vi "Kinect Analyze Particle.vi"(0 "Particle Mask In":T2, 5 "Extracted Mouse Image":T2, 7 "Height Threshold":dbl=100.0 format="%0.2f", 9 "Mouse Orientation":i32, 11 "error in":errorcluster) -> (4 "Mouse Data":T1, 15 "error out":errorcluster)   [LabVIEW 2011]
uses:
  <vilib>/vision/Image Controls.llb/IMAQ Image.ctl
  Mouse Data Cluster.ctl
  <vilib>/vision/NI_Vision_Development_Module.lvlib
panel:
  in  "Width of Band to \nCalculate Average Contour":i32=10
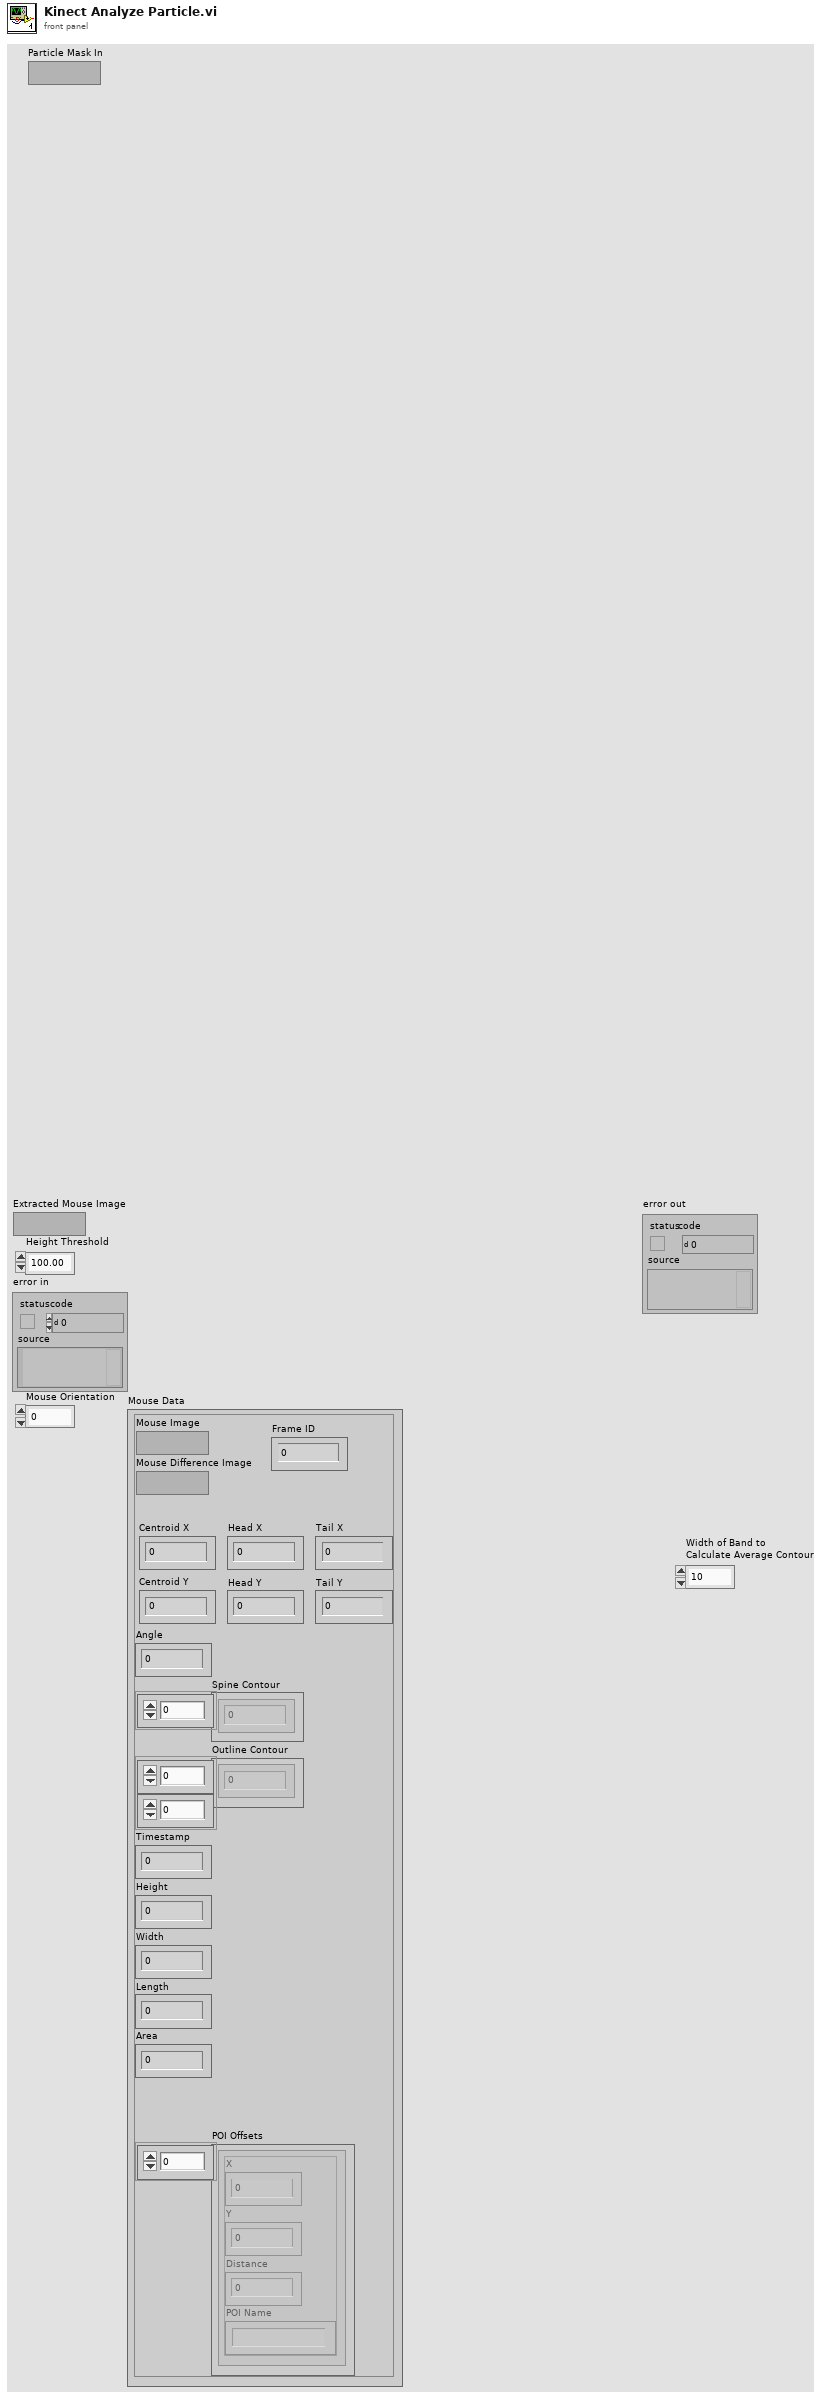
[diagram p1: front panel]
types:
  T1 = typedef "Mouse Data Cluster.ctl" = cluster{"Mouse Image":T2, "Mouse Difference Image":T2, "Angle":i32, "Spine Contour":i32[], "Outline Contour":i32[][], "Timestamp":dbl, "Height":i32, "Width":i32, "Length":i32, "Area":sgl, "POI Offsets":cluster{"X":i32, "Y":i32, "Distance":i32, "POI Name":string}[], "Frame ID":i16, "Centroid X":i32, "Centroid Y":i32, "Head X":i32, "Head Y":i32, "Tail X":i32, "Tail Y":i32}
  T2 = typedef "IMAQ Image.ctl" = refnum<image>
  T3 = typedef "Particle Parameters" = i32
  T4 = typedef "ROI Descriptor" = cluster{"Global Rectangle":i32[], "Contours":cluster{"ID":enum32{"External", "Internal"}, "Type":u32, "Coordinates":i32[]}[]}
  T5 = cluster{"ID":enum32{"External", "Internal"}, "Type":u32, "Coordinates":i32[]}[]
  T6 = cluster{"ID":enum32{"External", "Internal"}, "Type":u32, "Coordinates":i32[]}
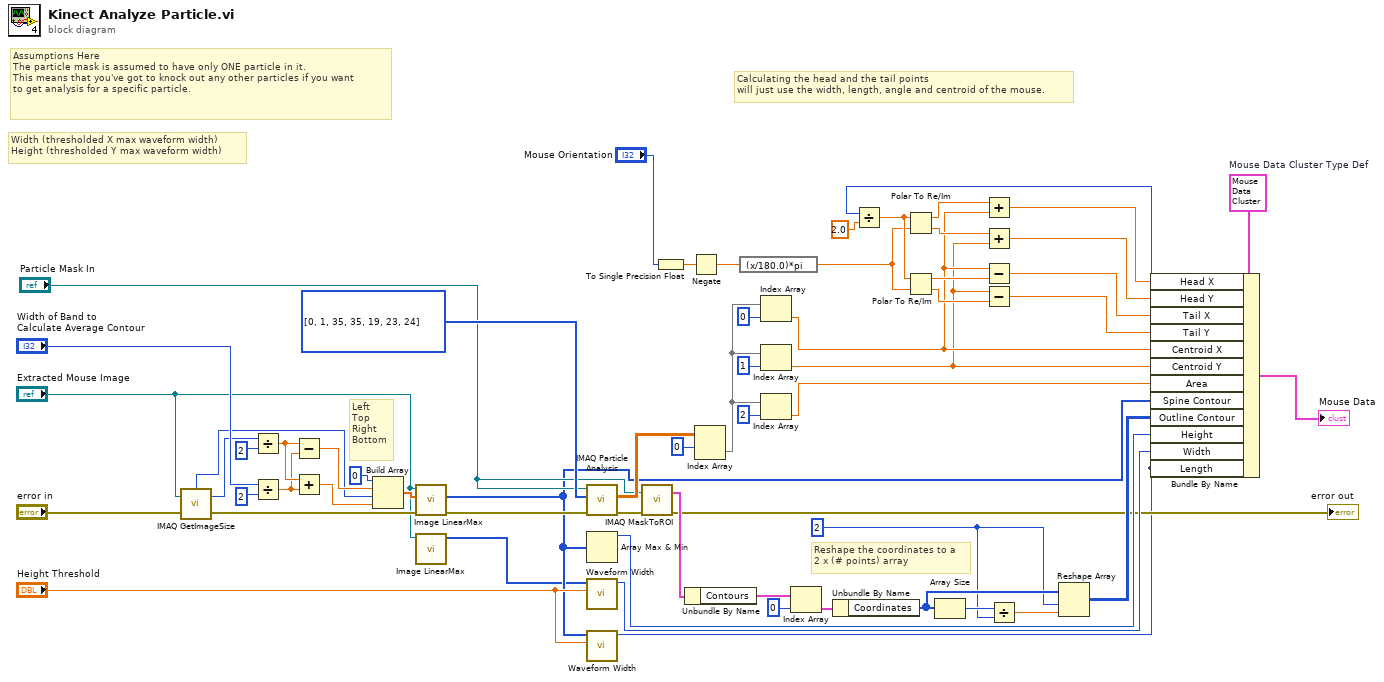
[diagram p0: block diagram]
diagram:
  w19 = T1 {"Mouse Image"=refnum, "Mouse Difference Image"=refnum, "Angle"=0, "Spine Contour"=[], "Outline Contour"=[], "Timestamp"=0.0, "Height"=0, "Width"=0, "Length"=0, "Area"=0.0, "POI Offsets"=[], "Frame ID"=0, "Centroid X"=0, "Centroid Y"=0, "Head X"=0, "Head Y"=0, "Tail X"=0, "Tail Y"=0}  # Mouse Data Cluster Type Def
  w31 = 2
  w54 = T3[] [0, 1, 35, 35, 19, 23, 24] items=["Center of Mass X", "Center of Mass Y", "First Pixel X", "First Pixel Y", "Bounding Rect Left", "Bounding Rect Top", "Bounding Rect Right", "Bounding Rect Bottom", "Max Feret Diameter Start X", "Max Feret Diameter Start Y", "Max Feret Diameter End X", "Max Feret Diameter End Y", "Max Horiz. Segment Length Left", "Max Horiz. Segment Length Right", "Max Horiz. Segment Length Row", "-", "Bounding Rect Width", "Bounding Rect Height", "Bounding Rect Diagonal", "Perimeter", "Convex Hull Perimeter", "Holes' Perimeter", "Max Feret Diameter", "Equivalent Ellipse Major Axis", "Equivalent Ellipse Minor Axis", "Equivalent Ellipse Minor Axis (Feret)", "Equivalent Rect Long Side", "Equivalent Rect Short Side", "Equivalent Rect Diagonal", "Equivalent Rect Short Side (Feret)", "Average Horiz. Segment Length", "Average Vert. Segment Length", "Hydraulic Radius", "Waddel Disk Diameter", "-", "Area", "Holes' Area", "Particle & Holes' Area", "Convex Hull Area", "Image Area", "-", "Number of Holes", "Number of Horiz. Segments", "Number of Vert. Segments", "-", "Orientation", "Max Feret Diameter Orientation", "-", "% Area/Image Area", "% Area/(Particle & Holes' Area)", "Ratio of Equivalent Ellipse Axes", "Ratio of Equivalent Rect Sides", "-", "Elongation Factor", "Compactness Factor", "Heywood Circularity Factor", "Type Factor", "-", "Sum X", "Sum Y", "Sum XX", "Sum XY", "Sum YY", "Sum XXX", "Sum XXY", "Sum XYY", "Sum YYY", "-", "Moment of Inertia XX", "Moment of Inertia XY", "Moment of Inertia YY", "Moment of Inertia XXX", "Moment of Inertia XXY", "Moment of Inertia XYY", "Moment of Inertia YYY", "Norm. Moment of Inertia XX", "Norm. Moment of Inertia XY", "Norm. Moment of Inertia YY", "Norm. Moment of Inertia XXX", "Norm. Moment of Inertia XXY", "Norm. Moment of Inertia XYY", "Norm. Moment of Inertia YYY", "Hu Moment 1", "Hu Moment 2", "Hu Moment 3", "Hu Moment 4", "Hu Moment 5", "Hu Moment 6", "Hu Moment 7"] ("Pixel Measurements")
  # "Calculating the head and the tail points\nwill just use the width, length, angle and centroid of the mouse."
  # "Reshape the coordinates to a \n2 x (# points) array"
  # "Assumptions Here\nThe particle mask is assumed to have only ONE particle in it.\nThis means that you've got to knock out any other particles if you want\nto get analysis for a specific particle."
  # "Width (thresholded X max waveform width)\nHeight (thresholded Y max waveform width)"
  # "Left\nTop\nRight\nBottom"
  n1 = call "IMAQ GetImageSize"("Image"="Extracted Mouse Image", "error in (no error)"="error in") -> ("Y Resolution"=w42:i32, "X Resolution"=w43:i32, "error out"=w26:errorcluster)  [unwired: 2 in]
  n2 = Divide(x=w42, y=2) -> (x/y=w46:dbl)
  n3 = Divide(x="Width of Band to \nCalculate Average Contour", y=2) -> (x/y=w45:dbl)
  n4 = Subtract(x=w46, y=w45) -> (x-y=w48:dbl)
  n5 = Add(x=w46, y=w45) -> (x+y=w47:dbl)
  n6 = Build Array(0 ("element"), w48, w43, w47) -> (w41:dbl[])
  n7 = call "Image LinearMax.vi"("error in (no error)"=w26, "Optional Rectangle"=w41, "Image Src"="Extracted Mouse Image") -> ("error out"=w25:errorcluster, "X Max"=w22:i16[])  [unwired: 6 in, 1 out]
  n8 = call "Image LinearMax.vi"("Image Src"="Extracted Mouse Image") -> ("Y Max"=w20:i16[])  [unwired: 8 in, 2 out]
  n9 = call "IMAQ Particle Analysis"("error in (no error)"=w25, "Pixel Measurements"=w54, "Image"="Particle Mask In") -> ("error out"=w24:errorcluster, "Particle Measurements (Pixels)"=w55:dbl[][])  [unwired: 3 in, 4 out]
  n10 = Array Max & Min(array=w22) -> (max value=w40:i16)  [unwired: 3 out]
  n11 = call "Waveform Width.vi"("Threshold"="Height Threshold", "Waveform"=w20) -> ("Width (in samples)"=w28:i32)  [unwired: 9 in]
  n12 = call "Waveform Width.vi"("Threshold"="Height Threshold", "Waveform"=w22) -> ("Width (in samples)"=w16:i32)  [unwired: 9 in]
  n13 = call "IMAQ MaskToROI"("Image"="Particle Mask In", "error in (no error)"=w24) -> ("ROI Descriptor"=w38:T4, "error out"=→"error out":errorcluster)  [unwired: 5 in, 1 out]
  n14 = To Single Precision Float(number="Mouse Orientation") -> (single precision float=w2:sgl)
  n15 = Unbundle By Name(w38) -> ("Contours"=w37:T5)
  n16 = Negate(x=w2) -> (-x=w4:sgl)
  n17 = Index Array(array=w55, index (row)=0) -> (element=w44:dbl[])  [unwired: 1 in]
  n18 = expression code="(x/180.0)*pi" ("degrees to radians")(w4) -> (w3:sgl)
  n19 = Index Array(array=w44, index=0) -> (element=w6:dbl)
  n20 = Index Array(array=w44, index=1) -> (element=w5:dbl)
  n21 = Index Array(array=w44, index=2) -> (element=w53:dbl)
  n22 = Index Array(array=w37, index=0) -> (element=w35:T6)
  n23 = Unbundle By Name(w35) -> ("Coordinates"=w34:i32[])
  n24 = Divide(x=w16, y=2.0) -> (x/y=w9:dbl)
  n25 = Polar To Re/Im(2:w3, 3:w9) -> (0:w14:dbl, 1:w15:dbl)
  n26 = Polar To Re/Im(2:w3, 3:w9) -> (0:w7:dbl, 1:w8:dbl)
  n27 = Array Size(array=w34) -> (size(s)=w32:i32)
  n28 = Add(x=w15, y=w6) -> (x+y=w13:dbl)
  n29 = Add(x=w14, y=w5) -> (x+y=w12:dbl)
  n30 = Subtract(x=w6, y=w8) -> (x-y=w11:dbl)
  n31 = Subtract(x=w5, y=w7) -> (x-y=w10:dbl)
  n32 = Divide(x=w32, y=w31) -> (x/y=w33:dbl)
  n33 = Reshape Array(w34, w31, w33) -> (w30:i32[][])
  n34 = Bundle By Name(cluster=w19, "Head X"=w13, "Head Y"=w12, "Tail X"=w11, "Tail Y"=w10, "Centroid X"=w6, "Centroid Y"=w5, "Area"=w53, "Spine Contour"=w22, "Outline Contour"=w30, "Height"=w40, "Width"=w28, "Length"=w16) -> (→"Mouse Data":T1)
